vi "IRH3T_PrinsFIFO.vi"(8 "error in (no error)":errorcluster, 9 "Initial Tardiness":u16, 10 "Schedule 2B Improved":u16[](array[numeric]), 11 "OSSP_Problem.lvclass":refnum<class "OSSP_Problem.lvclass">) -> (0 "error out":errorcluster, 1 "IRH3T (Reordered) Schedule Out":u16[](array[numeric]), 2 "IRH3T Schedule Out":u16[](array[numeric]), 3 "OSSP_Problem out":refnum<class "OSSP_Problem.lvclass">, 5 "Total Tardiness":u16)   [LabVIEW 2013, in "Scheduler.lvclass"]
uses:
  Scheduler.lvclass
  OSSP_Problem.lvclass
  OSSP_Problem.lvclass/OSSP_Problem.ctl
  UpdateMachineGaps.vi
  UpdateJobGaps.vi
  Find Intersecting Gaps.vi
  Transform to Plain Job and Machine Gaps Array.vi
panel:
  out "String":string="Total Tardiness has been improved. Total Tardiness is now %d"
  out "Job Completion Times":u16[](array[numeric])
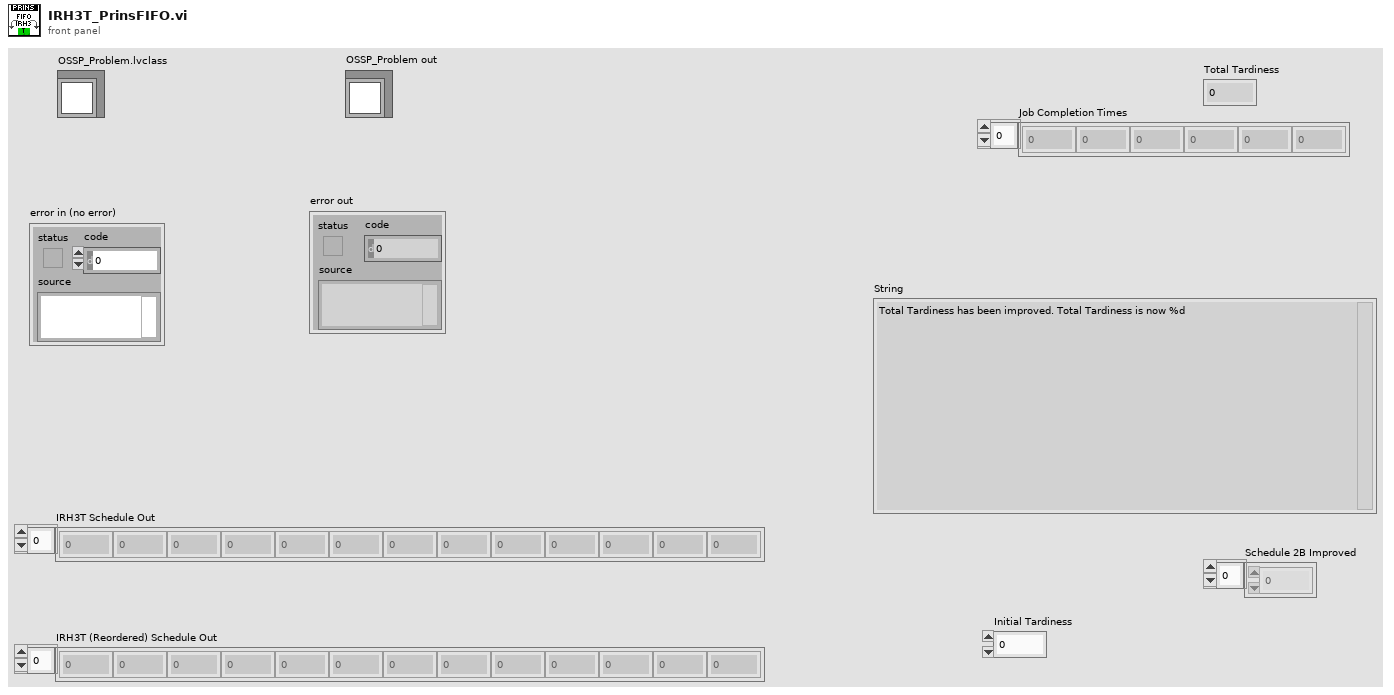
[diagram p1: front panel]
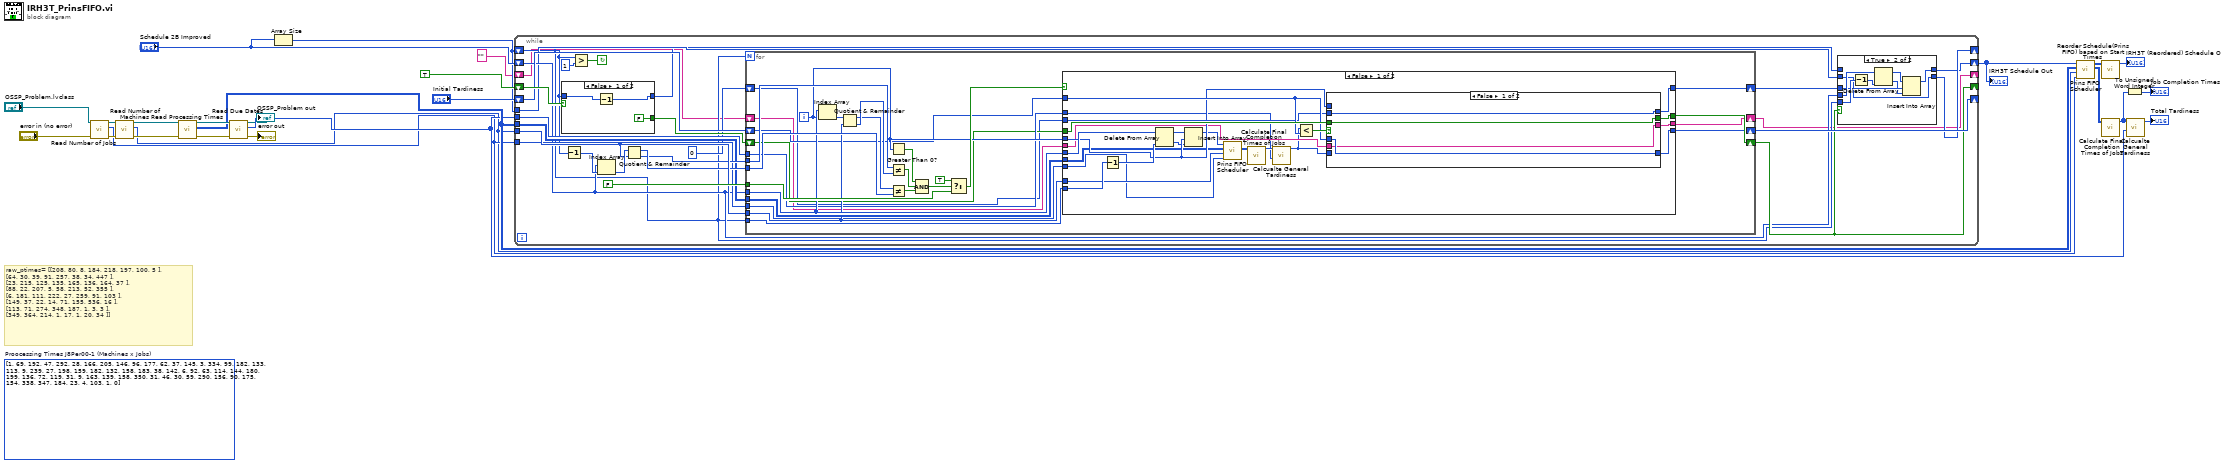
[diagram p0: block diagram]
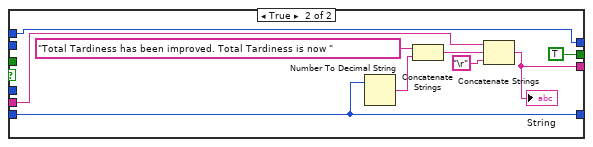
[diagram p3: hidden frame]
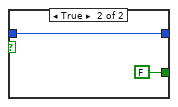
[diagram p5: hidden frame]
diagram:
  (unwired) u16[][] [[1, 69, 192, 47, 292, 28, 166, 205], [146, 96, 177, 62, 37, 145, 3, 334], [99, 182, 133, 113, 9, 239, 27, 198], [159, 182, 132, 158, 183, 38, 142, 6], [92, 63, 114, 144, 180, 199, 136, 72], [119, 31, 9, 163, 139, 158, 350, 31], [46, 30, 59, 290, 156, 90, 175, 154], [338, 347, 184, 23, 4, 103, 1, 0]]  # Proocessing Times J8Per00-1 (Machines x Jobs)
  # "raw_ptimes= [[208, 80, 8, 184, 218, 197, 100, 5 ],\n[64, 30, 39, 91, 257, 38, 34, 447 ],\n[23, 215, 125, 135, 165, 136, 164, 37 ],\n[88, 22, 207, 5, 58, 213, 52, 355 ],\n[6, 181, 111, 222, 27, 259, 91, 103 ],\n[149, 37, 22, 14, 71, 155, 536, 16 ],\n[113, 71, 274, 348, 187, 1, 3, 3 ],\n[349, 364, 214, 1, 17, 1, 20, 34 ]]"
  n1 = call "Read Number of Jobs.vi"("error in (no error)"="error in (no error)", "OSSP_Problem in"="OSSP_Problem.lvclass") -> ("error out"=w10:errorcluster, "Number of Jobs"=w5:i32, "OSSP_Problem out"=w13:refnum<class "OSSP_Problem.lvclass">)  [unwired: 7 in]
  n2 = call "Read Number of Machines.vi"("error in (no error)"=w10, "OSSP_Problem in"=w13) -> ("error out"=w9:errorcluster, "Number of Machines"=w4:i32, "OSSP_Problem out"=w12:refnum<class "OSSP_Problem.lvclass">)  [unwired: 7 in]
  n3 = call "Read Processing Times.vi"("error in (no error)"=w9, "OSSP_Problem in"=w12) -> ("error out"=w8:errorcluster, "Processing Times"=w7:u16[][], "OSSP_Problem out"=w11:refnum<class "OSSP_Problem.lvclass">)  [unwired: 7 in]
  n4 = call "Read Due Dates.vi"("error in (no error)"=w8, "OSSP_Problem in"=w11) -> ("error out"=→"error out":errorcluster, "Due Dates"=w6:u16[], "OSSP_Problem out"=→"OSSP_Problem out":refnum<class "OSSP_Problem.lvclass">)  [unwired: 7 in]
  n5 = Array Size(array="Schedule 2B Improved") -> (size(s)=w23:i32)
  n6 = while {
    shift-right: [w32] -> _
    shift-left: w23 -> [w30]
    shift-right: [w36] -> _
    shift-left: TRUE -> [w50]
    tunnel: w4 -> [w46]
    tunnel: w7 -> [w43]
    tunnel: w5 -> [w42]
    tunnel: w6 -> [w41]
    shift-right: [w38] -> _
    shift-left: "Initial Tardiness" -> [w40]
    shift-right: [w29] -> w21
    shift-left: "Schedule 2B Improved" -> [w35]
    tunnel: w23 -> [w33]
    shift-right: [w27] -> _
    shift-left: "" -> [w28]
    stop <- w51 continue-if-true
    n7 = case shown="False" w50 {
      tunnel: w30 -> [w132 w134]
      tunnel: [w131 w134] -> w31
      tunnel: [FALSE FALSE] -> w39
      frame False {
        n8 = Decrement(x=w132) -> (x-1=w131:i32)
      }
      frame True {
      }
    }
    n9 = Decrement(x=w30) -> (x-1=w49:i32)
    n10 = Greater?(x=w30, y=1) -> (0:w51:bool)
    n11 = Index Array(array=w35, index=w49) -> (element=w48:u16)
    n12 = Quotient & Remainder(x=w48, y=w46) -> (x-y*floor(x/y)=w45:i32, floor(x/y)=w44:i32)
    n13 = for {
      N: w30 -> [_]
      tunnel: FALSE -> [w80]
      tunnel: w35 -> [w77]
      tunnel: w46 -> [w73]
      tunnel: w45 -> [w83]
      tunnel: w44 -> [w87]
      tunnel: w30 -> [w76]
      tunnel: w43 -> [w74]
      tunnel: w42 -> [w72]
      tunnel: w41 -> [w71]
      shift-right: [w68] -> w36
      shift-left: w39 -> [w69]
      shift-right: [w67] -> w38
      shift-left: w40 -> [w70]
      shift-right: [w65] -> w34
      shift-left: 0 -> [w66]
      shift-right: [w63] -> w27
      shift-left: w28 -> [w64]
      i -> [w75]
      n14 = Index Array(array=w77, index=w75) -> (element=w89:u16)
      n15 = Quotient & Remainder(x=w89, y=w73) -> (x-y*floor(x/y)=w84:i32, floor(x/y)=w86:i32)
      n16 = Greater Than 0?(x=w75) -> (x > 0?=w88:bool)
      n17 = Not Equal?(x=w87, y=w86) -> (x != y?=w85:bool)
      n18 = Not Equal?(x=w84, y=w83) -> (x != y?=w82:bool)
      n19 = Compound Arithmetic op=AND(w88, w85, w82) -> (w81:bool)
      n20 = Select(t=TRUE, s=w81, f=w80) -> (s? t:f=w78:bool)
      n21 = case shown="False" w78 {
        tunnel: w77 -> [w112 _]
        tunnel: w76 -> [w111 _]
        tunnel: w75 -> [w101 _]
        tunnel: w74 -> [w95 _]
        tunnel: w73 -> [w94 _]
        tunnel: w72 -> [w93 _]
        tunnel: w71 -> [w91 _]
        tunnel: w70 -> [w104 w128]
        tunnel: w69 -> [w107 w129]
        tunnel: [w106 w129] -> w68
        tunnel: [w105 w128] -> w67
        tunnel: w66 -> [w103 w127]
        tunnel: [w102 w127] -> w65
        tunnel: w64 -> [w100 w126]
        tunnel: [w99 w126] -> w63
        frame False {
          n22 = Decrement(x=w111) -> (x-1=w110:i32)
          n23 = Delete From Array(array=w112, index=w110) -> (deleted portion=w98:u16, array with subset deleted=w109:u16[])  [unwired: 1 in]
          n24 = Insert Into Array(array=w109, index=w101, new element=w98) -> (w96:u16[])
          n25 = call "Prins FIFO Scheduler.vi"("Number of Jobs"=w93, "Number of Machines"=w94, "Processing Times(MxJ)"=w95, "Schedule In"=w96) -> ("Completion Times (MxJ)"=w97:i32[][])  [unwired: 6 in, 1 out]
          n26 = call "Calculate Final Completion Times of Jobs.vi"("Completion Times (MxJ)"=w97) -> ("Job Completion Times"=w92:i32[])  [unwired: 10 in]
          n27 = call "Calcualte General Tardiness.vi"("Due Dates"=w91, "Job Completion Times"=w92) -> ("Total Tardiness (U16)"=w90:u16)  [unwired: 9 in]
          n28 = Less?(x=w90, y=w104) -> (x < y?=w108:bool)
          n29 = case shown="False" w108 {
            tunnel: [w116 TRUE] -> w106
            tunnel: w107 -> [w116 _]
            tunnel: w90 -> [_ w123]
            tunnel: [w115 w123] -> w105
            tunnel: w104 -> [w115 _]
            tunnel: w103 -> [w114 _]
            tunnel: [w114 w124] -> w102
            tunnel: w101 -> [_ w124]
            tunnel: w100 -> [w113 w120]
            tunnel: [w113 w117] -> w99
            frame False {
            }
            frame True {
              n30 = Number To Decimal String(number=w123) -> (decimal integer string=w122:string)  [unwired: 1 in]
              n31 = Concatenate Strings("Total Tardiness has been improved. Total Tardiness is now ", w122) -> (w119:string)
              n32 = Concatenate Strings(w120, w119, "\r") -> (w117:string)
              "String" <- w117
            }
          }
        }
        frame True {
        }
      }
    }
    n33 = case shown="True" w36 {
      tunnel: w35 -> [w53 w62]
      tunnel: w30 -> [_ w60]
      tunnel: w34 -> [_ w58]
      tunnel: [w54 w56] -> w32
      tunnel: w33 -> [_ w56]
      tunnel: w31 -> [w54 _]
      tunnel: [w53 w55] -> w29
      frame False {
      }
      frame True {
        n34 = Decrement(x=w60) -> (x-1=w61:i32)
        n35 = Delete From Array(array=w62, index=w61) -> (deleted portion=w57:u16, array with subset deleted=w59:u16[])  [unwired: 1 in]
        n36 = Insert Into Array(array=w59, index=w58, new element=w57) -> (w55:u16[])
      }
    }
  }
  "IRH3T Schedule Out" <- w21
  n37 = call "Prins FIFO Scheduler.vi"("Number of Jobs"=w5, "Number of Machines"=w4, "Processing Times(MxJ)"=w7, "Schedule In"=w21) -> ("Completion Times (MxJ)"=w20:i32[][], "Start Times (MxJ)"=w16:i32[][])  [unwired: 6 in]
  n38 = call "Reorder Schedule(Prins FIFO) based on Start Times.vi"("Start Times (MxJ)"=w16) -> ("Reordered Schedule(Prins FIFO)"=→"IRH3T (Reordered) Schedule Out":u16[])  [unwired: 10 in]
  n39 = call "Calculate Final Completion Times of Jobs.vi"("Completion Times (MxJ)"=w20) -> ("Job Completion Times"=w18:i32[])  [unwired: 10 in]
  n40 = To Unsigned Word Integer(number=w18) -> (unsigned 16bit integer=→"Job Completion Times":u16[])
  n41 = call "Calcualte General Tardiness.vi"("Due Dates"=w6, "Job Completion Times"=w18) -> ("Total Tardiness (U16)"=→"Total Tardiness":u16)  [unwired: 9 in]
